vi "Untitlegd 1.vi"() -> ()   [LabVIEW 2015]
panel:
  in  "Tank 3":dbl(slide) scale=0.0..10.0
  in  "Tank 2":dbl(slide) scale=0.0..10.0
  in  "Tank":dbl(slide) scale=0.0..10.0
  out "Boolean 3":bool
  out "Boolean 2":bool
  out "Boolean":bool
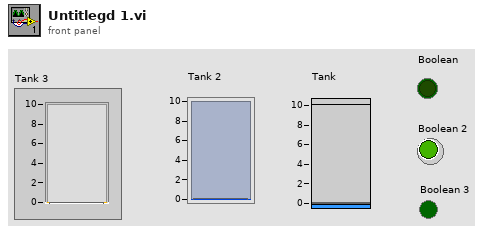
[diagram p1: front panel]
types:
  T1 = enum8{"Enabled", "Disabled", "Disabled and Grayed Out"}
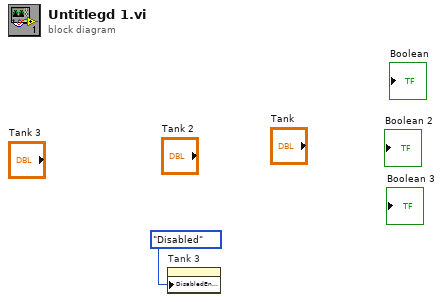
[diagram p0: block diagram]
diagram:
  n1 = property on="Tank 3" class="Slide (strict)"("DisabledEnum"=T1."Disabled" ("Disabled")) -> ()  [unwired: 2 in, 2 out]
